vi "CRC Check.vi"(0 "Command":string) -> (1 "CRC":u32, 2 "CRC Result":string)   [LabVIEW 2014, in "VISA.lvlib"]
uses:
  VISA.lvlib
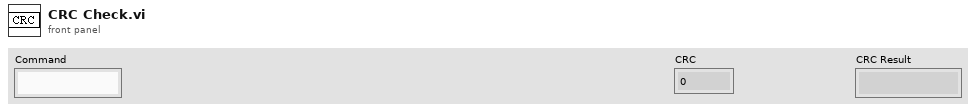
[diagram p1: front panel]
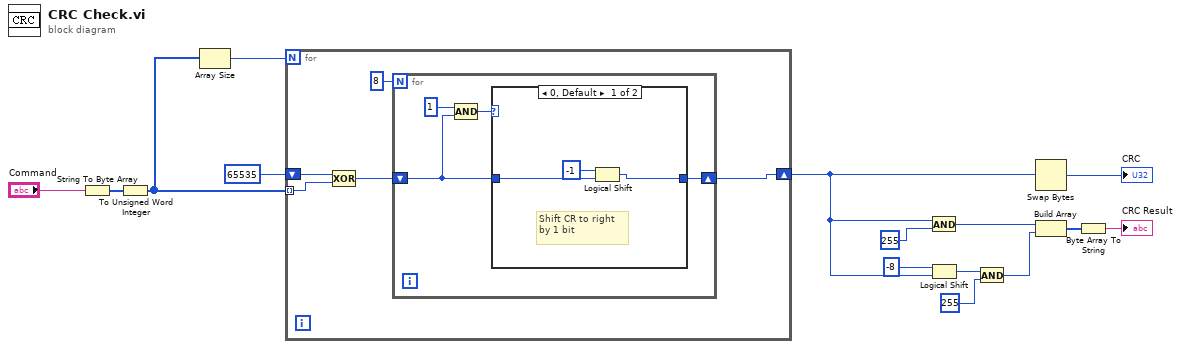
[diagram p0: block diagram]
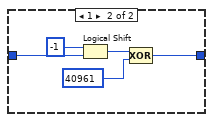
[diagram p2: hidden frame]
diagram:
  n1 = String To Byte Array(string="Command") -> (unsigned byte array=w14:u8[])
  n2 = To Unsigned Word Integer(number=w14) -> (unsigned 16bit integer=w2:u16[])
  n3 = Array Size(array=w2) -> (size(s)=w1:i32)
  n4 = for {
    N: w1 -> [_]
    shift-right: [w18] -> w9
    shift-left: u16 65535 -> [w19]
    tunnel: w2 -> [w17] mode=indexing
    n5 = Compound Arithmetic op=XOR(w19, w17) -> (w20:u32)
    n6 = for {
      N: 8 -> [_]
      shift-right: [w23] -> w18
      shift-left: w20 -> [w22]
      n7 = Compound Arithmetic op=AND(u16 1, w22) -> (w21:u32)
      n8 = case shown="0, Default" w21 {
        tunnel: [w26 w31] -> w23
        tunnel: w22 -> [w25 w28]
        frame 0, Default {
          # "Shift CR to right\nby 1 bit"
          n9 = Logical Shift(y=i16 -1, x=w25) -> (x << y=w26:u32)
        }
        frame 1 {
          n10 = Logical Shift(y=i16 -1, x=w28) -> (x << y=w30:u32)
          n11 = Compound Arithmetic op=XOR(w30, u32 40961) -> (w31:u32)
        }
      }
    }
  }
  n12 = And(x=w9, y=u16 255) -> (x .and. y?=w8:u32)
  n13 = Logical Shift(y=i16 -8, x=w9) -> (x << y=w11:u32)
  n14 = And(x=w11, y=u16 255) -> (x .and. y?=w7:u32)
  n15 = Swap Bytes(anything=w9) -> (byte swapped=→"CRC":u32)
  n16 = Build Array(w8, w7) -> (w6:u32[])
  n17 = Byte Array To String(unsigned byte array=w6) -> (string=→"CRC Result":string)
